vi "Create DataSet.vi"(8 "error in (no error)":errorcluster caption="错误输入（无错误）", 9 "DataGridView":refnum<k24>, 10 "dataSetName":string, 11 "DataSet 输入":refnum<class "DataSet.lvclass"> caption="DNL_LabVIEW Object in") -> (0 "error out":errorcluster caption="错误输出", 3 "DataSet 输出":refnum<class "DataSet.lvclass"> caption="DNL_LabVIEW Object out")   [LabVIEW 2012, in "Data Grid VIEW.lvlib" / "DataSet.lvclass"]
uses:
  DataSet.lvclass
  System.Windows.Forms
  System.Data
  DataSet.lvclass/DataSet.ctl
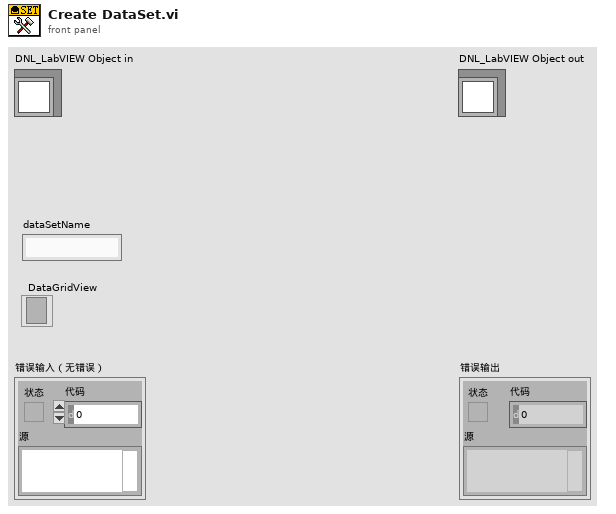
[diagram p1: front panel]
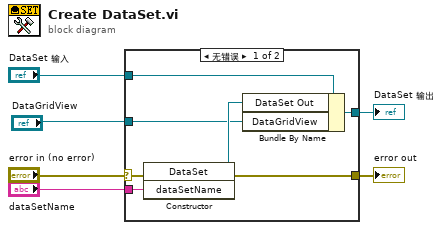
[diagram p0: block diagram]
diagram:
  n1 = case shown="无错误" "error in (no error)" {
    selector: "error in (no error)" -> [w9 w15]
    tunnel: [w8 w15] -> w5
    tunnel: [w10 w14] -> w3
    tunnel: "DataSet 输入" -> [w12 w14]
    tunnel: "dataSetName" -> [w13 _]
    tunnel: "DataGridView" -> [w7 _]
    frame No Error {
      n2 = constructor class="DataSet"(error in=w9, "dataSetName"=w13) -> (reference out=w11:refnum<k24>, error out=w8:errorcluster)  [unwired: 2 in, 2 out]
      n3 = Bundle By Name(cluster=w12, "DataSet Out"=w11, "DataGridView"=w7) -> (w10:refnum<class "DataSet.lvclass">)
    }
    frame Error {
    }
  }
  "error out" <- w5
  "DataSet 输出" <- w3
